vi "radiucenter2boundingbox.vi"(6 "Radius":i32, 7 "ycenter":i32, 8 "xcenter":i32) -> (0 "Bottom":i32, 2 "Right":i32, 3 "Top":i32, 5 "Left":i32)   [LabVIEW 2019]
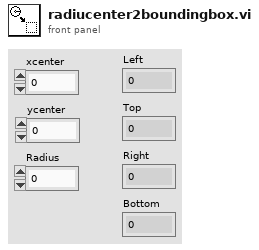
[diagram p1: front panel]
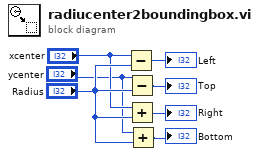
[diagram p0: block diagram]
diagram:
  n1 = Subtract(x="xcenter", y="Radius") -> (x-y=→"Left":i32)
  n2 = Subtract(x="ycenter", y="Radius") -> (x-y=→"Top":i32)
  n3 = Add(x="xcenter", y="Radius") -> (x+y=→"Right":i32)
  n4 = Add(x="ycenter", y="Radius") -> (x+y=→"Bottom":i32)
